vi "TDC_DAQV20_muon.vi"(8 "error in (no error)":errorcluster, 9 "stop":bool=TRUE, 10 "save data":bool=TRUE, 11 "SMA mode":bool=TRUE) -> (3 "rate":dbl)   [LabVIEW 2017]
uses:
  <vilib>/Utility/file.llb/Write Delimited Spreadsheet (DBL).vi
  <vilib>/Utility/file.llb/Write Delimited Spreadsheet (I64).vi
panel:
  out "substring 3":string
  out "hex integer string":string
  out "Year":string
  out "substring 2":string
  out "error out 3":errorcluster
  out "substring":string
  in  "factor":i32=128
  in  "displayCR":bool=TRUE
  in  "Counter Setting":dbl=100000.0 format="%#_13g"
  in  "replace dat":bool
  in  "append csv":bool=TRUE
  out "concatenated string":string
  out "number":u32=23
  out "element":string
  out "fine":u64=375 format="%x"
  in  "UDP Config":bool=TRUE
  in  "data  path":path=path "G:/tdc/2017"
  out "cal 2":u64[](graph)
  in  "Thresholds (mV)":u16[](array[numeric])=[580, 580, 580, 580, 600, 600, 600, 600, 580, 580, 600, 600, 600, 600, 600, 600, 580, 580, 600, 600, 600, 600, 600, 600, 580, 580, 600, 600, 600, 600, 600, 600]
  out "error out 2":errorcluster={"status"=TRUE, "code"=1, "source"="Dequeue Element in TDC_DAQV18_NewStructure.vi"}
  in  "display":bool=TRUE
  in  "Thresholds":u16=580
  in  "one key for threshold":bool=TRUE
  in  "RST":bool
  in  "通道数量":i32=64
  out "Cal Table":u32[](array[numeric])
  in  "channel for cal":i32
  out "channel number":u64
  in  "bytes to read":i32=320
  out "Calibration Counter":i32=100000
  out "Event index":i32=97959
  out "cal":u32[](graph)
  out "error out":errorcluster
  out "appended path":path=path "G:/tdc/2017/test_20240612_084516.dat"
  in  "filename":string="test"
  in  "Events":i32=110000 min=1
  in  "timeout (ms)":i32=10000
  in  "address":string="192.168.10.23"
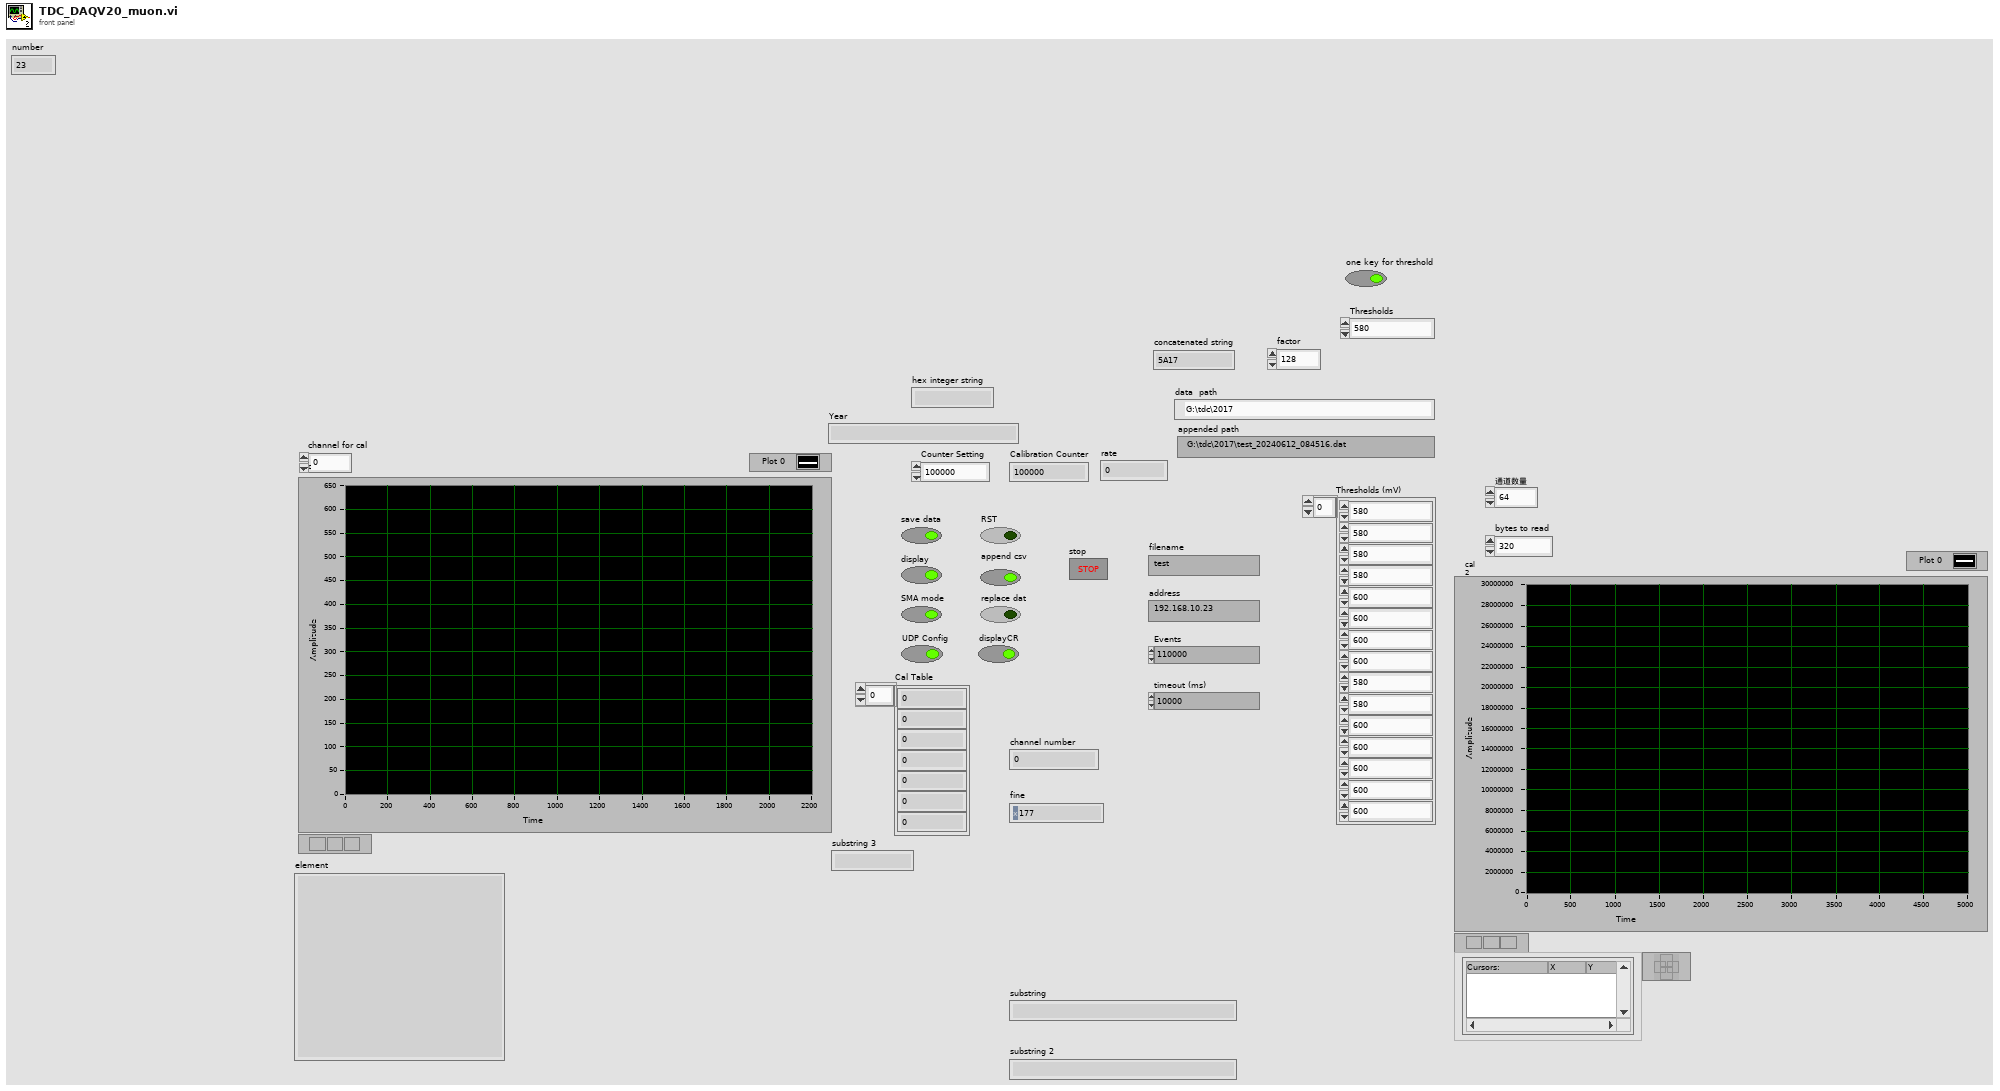
[diagram p1: front panel]
types:
  T1 = enum16{"open", "replace", "create", "open or create", "replace or create", "replace or create with confirmation"}
  T2 = enum16{"Standard", "Buffered", "CRLF", "Immediate"}
  T3 = enum16{"big-endian, network order", "native, host order", "little-endian"}
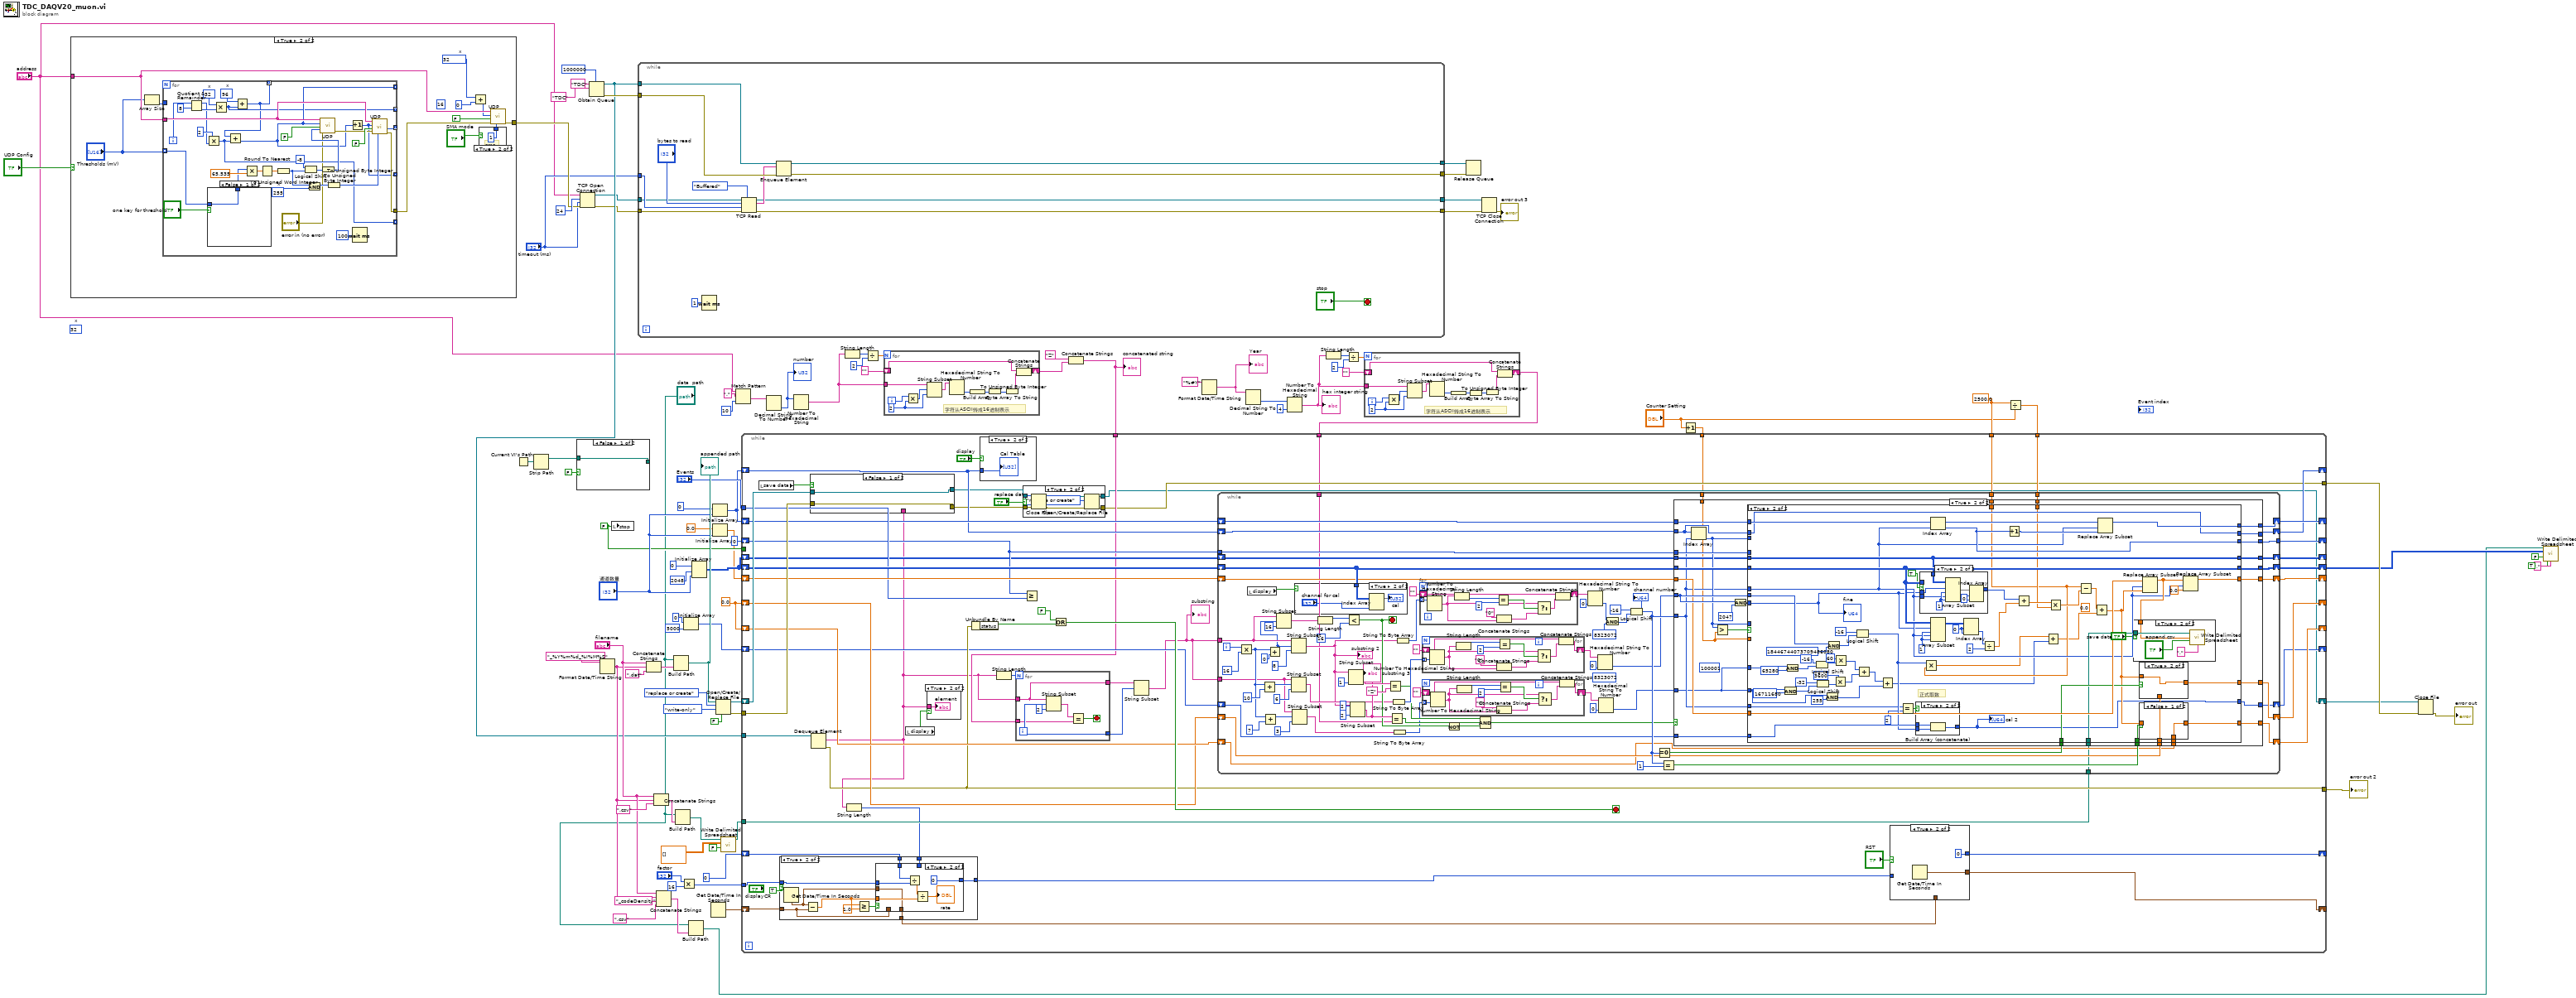
[diagram p0: block diagram]
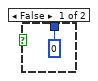
[diagram p3: hidden frame]
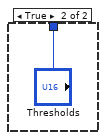
[diagram p4: hidden frame]
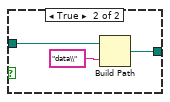
[diagram p5: hidden frame]
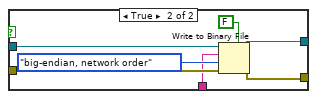
[diagram p7: hidden frame]
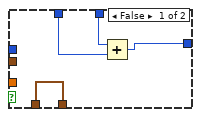
[diagram p10: hidden frame]
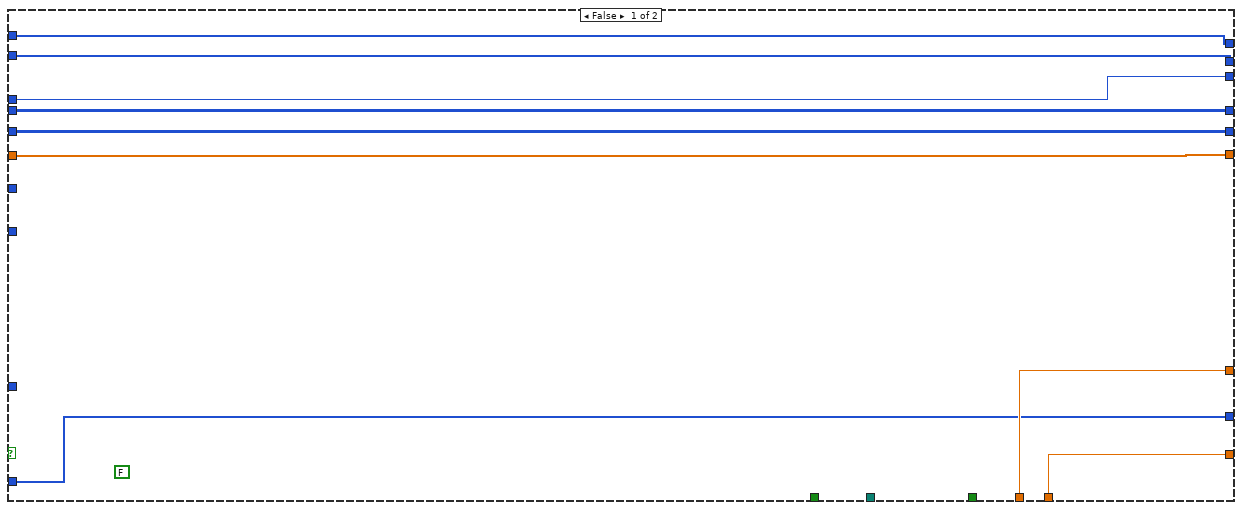
[diagram p14: hidden frame]
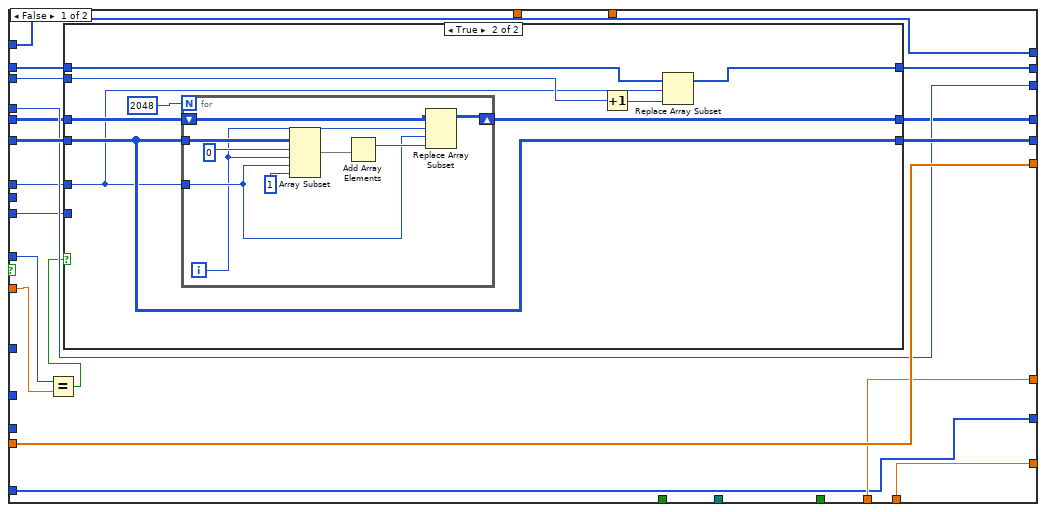
[diagram p15: hidden frame]
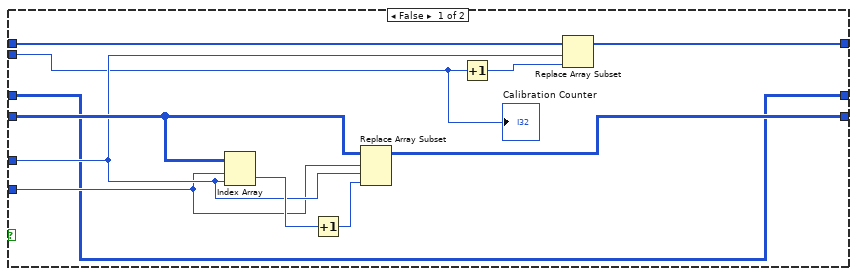
[diagram p16: hidden frame]
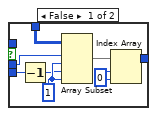
[diagram p19: hidden frame]
diagram:
  w20 = 2500.0 ("x")
  (unwired) u16 32  # x
  w64 = FALSE ("stop")
  w74 = 0.0
  n1 = case shown="True" "UDP Config" {
    tunnel: "address" -> [_ w107]
    tunnel: [_ w104] -> w65
    frame False {
    }
    frame True {
      (unwired) u32 16 ("Address")
      w98 = u16 32  # x
      n2 = Array Size(array="Thresholds (mV)") -> (size(s)=w101:i32)
      n3 = for {
        tunnel: w107 -> [w137]
        tunnel: "Thresholds (mV)" -> [w123] mode=indexing
        tunnel: [w131] -> _ mode=indexing
        tunnel: [w126] -> w105
        tunnel: w101 -> [_]
        tunnel: [w117] -> _ mode=indexing
        tunnel: [w116] -> _ mode=indexing
        tunnel: [w115] -> _ mode=indexing
        tunnel: [w114] -> _ mode=indexing
        tunnel: [w113] -> _ mode=indexing
        i -> [w118]
        w119 = u16 96  # x
        w120 = u16 32  # x
        w133 = u16 255  # x
        n4 = Quotient & Remainder(x=w118, y=8) -> (x-y*floor(x/y)=w112:i32, floor(x/y)=w121:i32)
        n5 = Multiply(x=2, y=w112) -> (x*y=w113:i32)
        n6 = case shown="False" "one key for threshold" {
          tunnel: [w143 "Thresholds"] -> w124
          tunnel: w123 -> [w143 _]
          frame False {
          }
          frame True {
          }
        }
        n7 = Multiply(x=w120, y=w121) -> (x*y=w115:i32)
        n8 = Add(x=w119, y=w115) -> (x+y=w114:i32)
        n9 = Add(x=w114, y=w113) -> (x+y=w117:i32)
        n10 = Multiply(x=w124, y=65.535) -> (x*y=w140:dbl)
        n11 = Round To Nearest(number=w140) -> (nearest integer value=w138:dbl)
        n12 = To Unsigned Word Integer(number=w138) -> (unsigned 16bit integer=w128:u16)
        n13 = Logical Shift(y=i16 -8, x=w128) -> (x << y=w135:u16)
        n14 = And(x=w128, y=w133) -> (x .and. y?=w132:u16)
        n15 = To Unsigned Byte Integer(number=w135) -> (unsigned 8bit integer=w134:u8)
        n16 = call "UDP.vi"("In"=w134, "error in (no error)"="error in (no error)", "Read (TRUE)"=FALSE, "Address"=w117, "IP address"=w137) -> ("error out"=w127:errorcluster)  [unwired: 4 in, 1 out]
        n17 = To Unsigned Byte Integer(number=w132) -> (unsigned 8bit integer=w130:u8)
        n18 = Increment(x=w117) -> (x+1=w116:i32)
        n19 = Wait (ms)(milliseconds to wait=u32 100) -> ()  [unwired: 1 out]
        n20 = call "UDP.vi"("In"=w130, "error in (no error)"=w127, "Read (TRUE)"=FALSE, "Address"=w116, "IP address"=w137) -> ("error out"=w126:errorcluster, "Out"=w131:u8)  [unwired: 4 in]
      }
      n21 = Add(x=w98, y=u32 0 ("Address")) -> (x+y=w97:u32)
      n22 = case shown="True" "SMA mode" {
        tunnel: [u8 0 ("In") u8 1 ("In")] -> w103
        frame False {
        }
        frame True {
          # "sma"
        }
      }
      n23 = call "UDP.vi"("In"=w103, "error in (no error)"=w105, "Read (TRUE)"=FALSE, "Address"=w97, "IP address"=w107) -> ("error out"=w104:errorcluster)  [unwired: 4 in, 1 out]
    }
  }
  n24 = Current VI's Path() -> (path=w90:path)
  n25 = Strip Path(path=w90) -> (stripped path=w89:path)  [unwired: 1 out]
  n26 = case shown="False" FALSE {
    tunnel: w89 -> [w145 w147]
    tunnel: [w145 w146] -> _
    frame False {
    }
    frame True {
      n27 = Build Path(base path=w147, name or relative path="data\\") -> (appended path=w146:path)
    }
  }
  n28 = TCP Open Connection(address="address", remote port or service name=u16 24 ("port"), timeout ms (60000)="timeout (ms)", error in (no error)=w65) -> (connection ID=w48:refnum<k5>, error out=w49:errorcluster)  [unwired: 1 in]
  n29 = Obtain Queue(max queue size (-1, unlimited)=1000000, name (unnamed)="TDC", element data type="TDC" ("name (unnamed)")) -> (queue out=w50:refnum<queue>, error out=w51:errorcluster)  [unwired: 2 in, 1 out]
  n30 = Format Date/Time String(time format string (%c)="_%Y%m%d_%I%M%S") -> (date/time string=w62:string)  [unwired: 2 in]
  n31 = local write "stop"(w64) -> ()
  n32 = while {
    tunnel: w50 -> [w162]
    tunnel: w51 -> [w161]
    tunnel: w49 -> [w159]
    tunnel: "timeout (ms)" -> [w158]
    tunnel: w48 -> [w157]
    tunnel: [w155] -> w47
    tunnel: [w154] -> w46
    tunnel: [w152] -> w45
    tunnel: [w151] -> w44
    stop <- "stop" stop-if-true
    n33 = Wait (ms)(milliseconds to wait=u32 1) -> ()  [unwired: 1 out]
    n34 = TCP Read(connection ID=w157, bytes to read="bytes to read", error in (no error)=w159, 7:T2."Buffered" ("mode (standard)"), 9:w158) -> (connection ID out=w155:refnum<k5>, data out=w156:string, error out=w154:errorcluster)
    n35 = Enqueue Element(queue=w162, element=w156, error in (no error)=w161) -> (queue out=w152:refnum<queue>, error out=w151:errorcluster)  [unwired: 1 in, 1 out]
  }
  n36 = Concatenate Strings("filename", w62, ".dat") -> (w88:string)
  n37 = Concatenate Strings("filename", w62, ".csv") -> (w76:string)
  n38 = Concatenate Strings("filename", w62, "_codeDensity" ("string"), ".csv") -> (w59:string)
  n39 = Build Path(base path="data  path", name or relative path=w88) -> (appended path=w87:path)
  "appended path" <- w87
  n40 = Build Path(base path="data  path", name or relative path=w76) -> (appended path=w71:path)
  n41 = Multiply(x="factor", y=16) -> (x*y=w13:i32)
  n42 = Initialize Array(u32 0 ("element"), 5000 ("dimension size")) -> (w38:u32[])
  n43 = Build Path(base path="data  path", name or relative path=w59) -> (appended path=w56:path)
  n44 = Initialize Array(u32 0 ("element"), 2048 ("dimension size"), "通道数量") -> (w73:u32[][])
  n45 = Get Date/Time In Seconds() -> (seconds since 1Jan1904=w66:timestamp)
  n46 = Initialize Array(u32 0 ("element"), "通道数量") -> (w75:u32[])
  n47 = Initialize Array(0.0, "通道数量") -> (w40:dbl[])
  n48 = Open/Create/Replace File(file path (use dialog)=w87, operation (0:open)=T1."replace or create", access (0:read/write)=enum16{"read/write", "read-only", "write-only"}."write-only", disable buffering (F)=FALSE) -> (refnum out=w92:refnum<file>, error out=w91:errorcluster)  [unwired: 2 in, 1 out]
  n49 = call-poly <vilib>:"Write Delimited Spreadsheet.vi"("file path (dialog if empty)"=w71, "2D data"=dbl[][] [], "append to file? (new file:F)"=FALSE) -> ("new file path (Not A Path if cancelled)"=w70:path)  [unwired: 11 in, 1 out]
  n50 = Match Pattern(string="address", regular expression="." ("search string"), offset (0)=10) -> (after substring=w27:string)  [unwired: 3 out]
  n51 = Decimal String To Number(string=w27) -> (number=w26:i32)  [unwired: 2 in, 1 out]
  "number" <- w26
  n52 = Number To Hexadecimal String(2:w26) -> (0:w24:string)  [unwired: 1 in]
  n53 = String Length(string=w24) -> (length=w32:i32)
  n54 = Divide(x=w32, y=2) -> (x/y=w33:dbl)
  n55 = for {
    N: w33 -> [_]
    shift-right: [w173] -> w23
    shift-left: "" ("format string") -> [w172]
    tunnel: w24 -> [w163]
    i -> [w171]
    w165 = 2 ("y")
    # "字符从ASCII转成16进制表示"
    n56 = Multiply(x=w171, y=w165) -> (x*y=w164:i32)
    n57 = String Subset(string=w163, offset (0)=w164, length (rest)=w165) -> (substring=w166:string)
    n58 = Hexadecimal String To Number(string=w166) -> (number=w170:u32)  [unwired: 2 in, 1 out]
    n59 = Build Array(w170) -> (w169:u32[])
    n60 = To Unsigned Byte Integer(number=w169) -> (unsigned 8bit integer=w168:u8[])
    n61 = Byte Array To String(unsigned byte array=w168) -> (string=w167:string)
    n62 = Concatenate Strings(w172, w167) -> (w173:string)
  }
  n63 = Concatenate Strings("Z", w23) -> (w22:string)
  "concatenated string" <- w22
  n64 = Format Date/Time String(time format string (%c)="%#Y") -> (date/time string=w9:string)  [unwired: 2 in]
  "Year" <- w9
  n65 = Decimal String To Number(string=w9) -> (number=w8:i32)  [unwired: 2 in, 1 out]
  n66 = Number To Hexadecimal String(1:i16 4 ("width (-)"), 2:w8) -> (0:w2:string)
  "hex integer string" <- w2
  n67 = String Length(string=w2) -> (length=w4:i32)
  n68 = Divide(x=w4, y=2) -> (x/y=w5:dbl)
  n69 = for {
    N: w5 -> [_]
    shift-right: [w184] -> w1
    shift-left: "" ("format string") -> [w183]
    tunnel: w2 -> [w174]
    i -> [w182]
    w176 = 2 ("y")
    # "字符从ASCII转成16进制表示"
    n70 = Multiply(x=w182, y=w176) -> (x*y=w175:i32)
    n71 = String Subset(string=w174, offset (0)=w175, length (rest)=w176) -> (substring=w177:string)
    n72 = Hexadecimal String To Number(string=w177) -> (number=w181:u32)  [unwired: 2 in, 1 out]
    n73 = Build Array(w181) -> (w180:u32[])
    n74 = To Unsigned Byte Integer(number=w180) -> (unsigned 8bit integer=w179:u8[])
    n75 = Byte Array To String(unsigned byte array=w179) -> (string=w178:string)
    n76 = Concatenate Strings(w183, w178) -> (w184:string)
  }
  n77 = Release Queue(queue=w45, error in (no error)=w44) -> ()  [unwired: 1 in, 3 out]
  n78 = TCP Close Connection(connection ID=w47, error in (no error)=w46) -> (error out=→"error out 3":errorcluster)  [unwired: 1 in, 1 out]
  n79 = Increment(x="Counter Setting") -> (x+1=w16:dbl)
  n80 = Divide(x=w20, y="Counter Setting") -> (x/y=w19:dbl)
  n81 = while {
    tunnel: w91 -> [w239]
    tunnel: [w213] -> w43
    tunnel: [w197] -> w84
    shift-right: [w236] -> w57
    shift-left: w73 -> [w237]
    shift-right: [w222] -> _
    shift-left: w40 -> [w235]
    tunnel: "Events" -> [w233]
    shift-right: [w232] -> _
    shift-left: w75 -> [w231]
    shift-right: [w230] -> _
    shift-left: u32 0 ("element") -> [w229]
    shift-right: [w228] -> _
    shift-left: w75 -> [w215]
    shift-right: [w227] -> _
    shift-left: w74 -> [w224]
    shift-right: [w226] -> _
    shift-left: w74 -> [w225]
    shift-right: [w217] -> _
    shift-left: w73 -> [w223]
    tunnel: w70 -> [w209]
    shift-right: [w221] -> _
    shift-left: 0 -> [w191]
    shift-right: [w219] -> _
    shift-left: w66 -> [w218]
    tunnel: w64 -> [_]
    tunnel: w50 -> [w214]
    shift-right: [w210] -> _
    shift-left: w38 -> [w211]
    tunnel: w22 -> [w205]
    tunnel: w20 -> [w203]
    tunnel: w19 -> [w202]
    shift-right: [w196] -> w18
    shift-left: w92 -> [w238]
    tunnel: w16 -> [w195]
    tunnel: w13 -> [w188]
    tunnel: w1 -> [w185]
    stop <- w234 stop-if-true
    n82 = local read "save data"() -> (w190:bool)
    n83 = Dequeue Element(queue=w214) -> (element=w201:string, error out=w213:errorcluster)  [unwired: 2 in, 2 out]
    n84 = case shown="False" w190 {
      tunnel: w239 -> [w241 w249]
      tunnel: w238 -> [w242 w248]
      tunnel: w201 -> [_ w245]
      tunnel: [w242 w244] -> w200
      tunnel: [w241 w243] -> w198
      frame False {
      }
      frame True {
        n85 = Write to Binary File(file (use dialog)=w248, data=w245, error in=w249, 5:FALSE ("prepend array or string size? (T)"), 9:T3."big-endian, network order" ("byte order (0:big-endian, network order)")) -> (refnum out=w244:refnum<file>, error out=w243:errorcluster)  [unwired: 1 in, 1 out]
      }
    }
    n86 = String Length(string=w201) -> (length=w192:i32)
    n87 = case shown="True" TRUE {
      tunnel: w218 -> [w266 w271]
      tunnel: [w266 w272] -> w194
      tunnel: w191 -> [w265 w270]
      tunnel: w192 -> [_ w269]
      tunnel: [w265 w268] -> w193
      tunnel: w188 -> [_ w267]
      frame False {
      }
      frame True {
        n88 = Get Date/Time In Seconds() -> (seconds since 1Jan1904=w273:timestamp)
        n89 = Subtract(x=w273, y=w271) -> (x-y=w275:dbl)
        n90 = Greater Or Equal?(x=w275, y=1.0) -> (x >= y?=w276:bool)
        n91 = case shown="True" w276 {
          tunnel: w275 -> [_ w287]
          tunnel: w273 -> [_ w285]
          tunnel: [w280 w285] -> w272
          tunnel: w271 -> [w280 _]
          tunnel: w270 -> [w279 w282]
          tunnel: w269 -> [w278 _]
          tunnel: [w277 0] -> w268
          tunnel: w267 -> [_ w281]
          frame False {
            n92 = Add(x=w278, y=w279) -> (x+y=w277:i32)
          }
          frame True {
            n93 = Divide(x=w282, y=w281) -> (x/y=w284:dbl)
            n94 = Divide(x=w284, y=w287) -> (x/y=→"rate":dbl)
          }
        }
      }
    }
    n95 = local read "display"() -> (w189:bool)
    n96 = case shown="True" w189 {
      tunnel: w201 -> [_ w240]
      frame False {
      }
      frame True {
        "element" <- w240
      }
    }
    n97 = Unbundle By Name(w213) -> ("status"=w212:bool)
    n98 = case shown="True" "display" {
      tunnel: w215 -> [_ w288]
      frame False {
      }
      frame True {
        "Cal Table" <- w288
      }
    }
    n99 = String Length(string=w201) -> (length=w208:i32)
    n100 = for {
      N: w208 -> [_]
      tunnel: w201 -> [w261]
      tunnel: [w261] -> w207
      tunnel: [w260] -> w206
      tunnel: w205 -> [w259]
      i -> [w260]
      stop <- w262 stop-if-true
      n101 = String Subset(string=w261, offset (0)=w260, length (rest)=2 ("length (rest)")) -> (substring=w263:string)
      n102 = Equal?(x=w263, y=w259) -> (x = y?=w262:bool)
    }
    n103 = case shown="True" "replace dat" {
      tunnel: w200 -> [w251 w257]
      tunnel: [w251 w256] -> w196
      tunnel: w198 -> [w250 w253]
      tunnel: [w250 w252] -> w197
      frame False {
      }
      frame True {
        n104 = Close File(refnum=w257, error in=w253) -> (path=w258:path, error out=w254:errorcluster)
        n105 = Open/Create/Replace File(file path (use dialog)=w258, error in=w254, operation (0:open)=T1."replace or create") -> (refnum out=w256:refnum<file>, error out=w252:errorcluster)  [unwired: 3 in, 1 out]
      }
    }
    n106 = Greater Or Equal?(x=w229, y=w233) -> ()  [unwired: 1 out]
    n107 = Or(x=FALSE, y=w212) -> (x .or. y?=w234:bool)
    n108 = String Subset(string=w207, offset (0)=w206) -> (substring=w186:string)  [unwired: 1 in]
    "substring" <- w186
    n109 = while {
      tunnel: w186 -> [w315]
      shift-right: [w366] -> w236
      shift-left: w237 -> [w364]
      shift-right: [w362] -> w222
      shift-left: w235 -> [w363]
      shift-right: [w357] -> w232
      shift-left: w231 -> [w356]
      tunnel: [w355] -> w230
      tunnel: w229 -> [w354]
      shift-right: [w352] -> w228
      shift-left: w215 -> [w353]
      shift-right: [w347] -> w227
      shift-left: w224 -> [w345]
      shift-right: [w343] -> w226
      shift-left: w225 -> [w344]
      tunnel: w209 -> [w342]
      shift-right: [w341] -> w217
      shift-left: w223 -> [w309]
      shift-right: [w338] -> w210
      shift-left: w211 -> [w339]
      tunnel: w186 -> [w301]
      tunnel: w203 -> [w317]
      tunnel: w202 -> [w316]
      tunnel: w195 -> [w308]
      tunnel: w185 -> [w293]
      i -> [w367]
      stop <- w311 stop-if-true
      (unwired) u64 8323072 ("port")
      n110 = Multiply(x=w367, y=16 ("length (rest)")) -> (x*y=w302:i32)
      n111 = local read "display"() -> (w340:bool)
      n112 = Add(x=w302, y=10 ("length (rest)")) -> (x+y=w330:i32)
      n113 = Add(x=w302, y=7 ("length (rest)")) -> (x+y=w304:i32)
      n114 = Add(x=w302, y=0 ("length (rest)")) -> (x+y=w314:i32)
      n115 = String Subset(string=w315, offset (0)=w314, length (rest)=16 ("y")) -> (substring=w312:string)
      n116 = String Subset(string=w315, offset (0)=w314, length (rest)=8 ("length (rest)")) -> (substring=w294:string)
      "substring 2" <- w294
      n117 = String Subset(string=w301, offset (0)=w330, length (rest)=6 ("length (rest)")) -> (substring=w307:string)
      n118 = String Subset(string=w301, offset (0)=w304, length (rest)=3 ("length (rest)")) -> (substring=w297:string)
      n119 = case shown="True" w340 {
        tunnel: w364 -> [_ w393]
        frame False {
        }
        frame True {
          n120 = Index Array(array=w393, index (col)="channel for cal") -> (element=→"cal":u32[])  [unwired: 1 in]
        }
      }
      n121 = String Length(string=w312) -> (length=w361:i32)
      n122 = Less?(x=w361, y=16) -> (x < y?=w311:bool)
      n123 = String Subset(string=w294, length (rest)=1 ("length (rest)")) -> (substring=w335:string)  [unwired: 1 in]
      n124 = String Subset(string=w294, offset (0)=2, length (rest)=2 ("length (rest)")) -> (substring=w318:string)
      "substring 3" <- w318
      n125 = Equal?(x=w335, y="Z" ("format string")) -> (x = y?=w320:bool)
      n126 = Equal?(x=w318, y=w293) -> (x = y?=w319:bool)
      n127 = String To Byte Array(string=w307) -> (unsigned byte array=w327:u8[])
      n128 = String To Byte Array(string=w297) -> (unsigned byte array=w296:u8[])
      n129 = String To Byte Array(string=w294) -> (unsigned byte array=w369:u8[])
      n130 = for {
        shift-right: [w581] -> w324
        shift-left: "" ("format string") -> [w578]
        tunnel: w369 -> [w582] mode=indexing
        n131 = Number To Hexadecimal String(2:w582) -> (0:w574:string)  [unwired: 1 in]
        n132 = String Length(string=w574) -> (length=w580:i32)
        n133 = Equal?(x=w580, y=2) -> (x = y?=w577:bool)
        n134 = Concatenate Strings("0" ("format string"), w574) -> (w576:string)
        n135 = Select(t=w574, s=w577, f=w576) -> (s? t:f=w573:string)
        n136 = Concatenate Strings(w578, w573) -> (w581:string)
      }
      n137 = for {
        shift-right: [w389] -> w325
        shift-left: "" ("format string") -> [w381]
        tunnel: w327 -> [w390] mode=indexing
        n138 = Number To Hexadecimal String(2:w390) -> (0:w383:string)  [unwired: 1 in]
        n139 = String Length(string=w383) -> (length=w388:i32)
        n140 = Concatenate Strings("0" ("format string"), w383) -> (w385:string)
        n141 = Equal?(x=w388, y=2) -> (x = y?=w386:bool)
        n142 = Select(t=w383, s=w386, f=w385) -> (s? t:f=w382:string)
        n143 = Concatenate Strings(w381, w382) -> (w389:string)
      }
      n144 = for {
        shift-right: [w379] -> w300
        shift-left: "" ("format string") -> [w371]
        tunnel: w296 -> [w380] mode=indexing
        n145 = Number To Hexadecimal String(2:w380) -> (0:w373:string)  [unwired: 1 in]
        n146 = String Length(string=w373) -> (length=w378:i32)
        n147 = Concatenate Strings("0" ("format string"), w373) -> (w375:string)
        n148 = Equal?(x=w378, y=2) -> (x = y?=w376:bool)
        n149 = Select(t=w373, s=w376, f=w375) -> (s? t:f=w372:string)
        n150 = Concatenate Strings(w371, w372) -> (w379:string)
      }
      n151 = Not(x=w311) -> (.not. x?=w310:bool)
      n152 = Compound Arithmetic op=AND(w320, w319, w310) -> (w333:bool)
      n153 = Hexadecimal String To Number(string=w324, default (0uL)=u64 0 ("default (0 U32)")) -> (number=w365:u64)  [unwired: 1 in, 1 out]
      n154 = Hexadecimal String To Number(string=w325, default (0uL)=u64 0 ("default (0 U32)")) -> (number=w323:u64)  [unwired: 1 in, 1 out]
      n155 = Hexadecimal String To Number(string=w300, default (0uL)=u64 0 ("default (0 U32)")) -> (number=w295:u64)  [unwired: 1 in, 1 out]
      n156 = And(x=w365, y=u64 8323072 ("port")) -> (x .and. y?=w358:u64)
      n157 = Logical Shift(y=i16 -16, x=w358) -> (x << y=w350:u64)
      "channel number" <- w350
      n158 = Equal To 0?(x=w350) -> (x = 0?=w348:bool)
      n159 = Equal?(x=w350, y=u64 1) -> (x = y?=w346:bool)
      n160 = case shown="True" w333 {
        tunnel: w323 -> [_ w433]
        tunnel: w354 -> [w399 w423]
        tunnel: w364 -> [w402 w432]
        tunnel: [w402 w431] -> w366
        tunnel: [w401 w428] -> w362
        tunnel: w363 -> [w401 w427]
        tunnel: w350 -> [_ w407]
        tunnel: w356 -> [w400 w426]
        tunnel: [w400 w425] -> w357
        tunnel: [w399 w424] -> w355
        tunnel: w353 -> [w398 w422]
        tunnel: [w398 w421] -> w352
        tunnel: w348 -> [_ w420]
        tunnel: w345 -> [w397 w419]
        tunnel: [w397 w418] -> w347
        tunnel: w346 -> [_ w417]
        tunnel: w344 -> [w396 w416]
        tunnel: [w396 w415] -> w343
        tunnel: w309 -> [w395 w413]
        tunnel: [w395 w412] -> w341
        tunnel: w342 -> [_ w411]
        tunnel: w339 -> [w394 w409]
        tunnel: [w394 w408] -> w338
        tunnel: w317 -> [_ w406]
        tunnel: w316 -> [_ w405]
        tunnel: w308 -> [_ w404]
        tunnel: w295 -> [_ w403]
        frame False {
          (unwired) FALSE
        }
        frame True {
          (unwired) 100001 ("y")
          n161 = Index Array(array=w422, index=w407) -> (element=w414:u32)
          n162 = Greater?(x=w414, y=w404) -> (0:w410:bool)
          n163 = And(x=w433, y=u64 2047 ("port")) -> (x .and. y?=w429:u64)
          n164 = case shown="True" w410 {
            tunnel: w433 -> [_ w545]
            tunnel: w432 -> [w451 w531]
            tunnel: [w450 w531] -> w431
            tunnel: w429 -> [w442 w504]
            tunnel: [w449 w515] -> w428
            tunnel: w427 -> [w449 w538]
            tunnel: w423 -> [w447 _]
            tunnel: w407 -> [w445 w513]
            tunnel: w426 -> [w448 w537]
            tunnel: [w448 w536] -> w425
            tunnel: [w447 w534] -> w424
            tunnel: w414 -> [w443 _]
            tunnel: w422 -> [w446 w533]
            tunnel: [w444 w533] -> w421
            tunnel: w420 -> [_ w526]
            tunnel: w419 -> [w441 w525]
            tunnel: [w441 w524] -> w418
            tunnel: w417 -> [_ w523]
            tunnel: w416 -> [w440 w522]
            tunnel: [w440 w521] -> w415
            tunnel: w414 -> [w438 _]
            tunnel: w404 -> [w435 _]
            tunnel: w413 -> [w437 w517]
            tunnel: [w436 w517] -> w412
            tunnel: w411 -> [_ w516]
            tunnel: w409 -> [w434 w510]
            tunnel: [w434 w508] -> w408
            tunnel: w407 -> [_ w505]
            tunnel: w406 -> [_ w502]
            tunnel: w405 -> [_ w503]
            tunnel: w403 -> [_ w497]
            tunnel: w403 -> [_ w485]
            frame False {
              n165 = Equal?(x=w438, y=w435) -> (x = y?=w439:bool)
              n166 = case shown="True" w439 {
                tunnel: w451 -> [w462 w468]
                tunnel: [w460 w468] -> w450
                tunnel: w446 -> [w458 w466]
                tunnel: w445 -> [w457 w463]
                tunnel: [w455 w465] -> w444
                tunnel: w443 -> [w454 w464]
                tunnel: w442 -> [w453 _]
                tunnel: w437 -> [w452 w470]
                tunnel: [w452 w469] -> w436
                frame False {
                  n167 = Index Array(array=w462, index (row)=w453, index (col)=w457) -> (element=w461:u32)
                  n168 = Increment(x=w461) -> (x+1=w459:u32)
                  n169 = Replace Array Subset(array=w462, new element=w459, index (row)=w453, index (col)=w457) -> (w460:u32[][])
                  n170 = Increment(x=w454) -> (x+1=w456:u32)
                  n171 = Replace Array Subset(array=w458, new element=w456, index=w457) -> (w455:u32[])
                  "Calibration Counter" <- w454
                }
                frame True {
                  n172 = for {
                    N: 2048 -> [_]
                    tunnel: w468 -> [w480]
                    tunnel: w463 -> [w473]
                    shift-right: [w475] -> w469
                    shift-left: w470 -> [w476]
                    i -> [w472]
                    n173 = Array Subset(array=w480, index (row)=0 ("索引"), length (row)=w472, index (col)=w473, length (col)=1 ("长度")) -> (w477:u32[][])
                    n174 = Add Array Elements(numeric array=w477) -> (sum=w474:u32)
                    n175 = Replace Array Subset(array=w476, new element=w474, index (row)=w472, index (col)=w473) -> (w475:u32[][])
                  }
                  n176 = Increment(x=w464) -> (x+1=w467:u32)
                  n177 = Replace Array Subset(array=w466, new element=w467, index=w463) -> (w465:u32[])
                }
              }
            }
            frame True {
              (unwired) 0.0 ("x")
              w528 = 0 ("索引 (行)")
              w530 = 1 ("长度")
              # "正式取数"
              n178 = And(x=w485, y=u64 16711680 ("port")) -> (x .and. y?=w494:u64)
              n179 = And(x=w497, y=u64 65280 ("port")) -> (x .and. y?=w500:u64)
              n180 = Logical Shift(y=i16 -16, x=w500) -> (x << y=w491:u64)
              n181 = Logical Shift(y=i16 -32, x=w494) -> (x << y=w493:u64)
              n182 = And(x=w485, y=u64 255 ("port")) -> (x .and. y?=w484:u64)
              n183 = And(x=w545, y=u64 18446744073709486080 ("port")) -> (x .and. y?=w542:u64)
              n184 = Multiply(x=u64 3600, y=w493) -> (x*y=w488:u64)
              n185 = Multiply(x=u64 60, y=w491) -> (x*y=w489:u64)
              n186 = Logical Shift(y=i16 -16, x=w542) -> (x << y=w509:u64)
              n187 = Add(x=w489, y=w488) -> (x+y=w487:u64)
              n188 = Add(x=w487, y=w484) -> (x+y=w481:u64)
              n189 = Equal?(x=w505, y=u32 2) -> (x = y?=w507:bool)
              n190 = case shown="True" w507 {
                tunnel: w510 -> [w546 w549]
                tunnel: w509 -> [_ w548]
                tunnel: [w546 w547] -> w508
                frame False {
                }
                frame True {
                  n191 = Build Array (concatenate)(w549, w548) -> (w547:u64[])
                }
              }
              "cal 2" <- w508
              n192 = case shown="True" TRUE {
                tunnel: [w556 w564] -> w540
                tunnel: w531 -> [_ _]
                tunnel: w513 -> [w561 w562]
                tunnel: w504 -> [w559 w567]
                tunnel: w517 -> [w560 w568]
                frame False {
                  w555 = 0 ("index (row)")
                  w558 = 1 ("长度")
                  n193 = Decrement(x=w561) -> (x-1=w554:u64)
                  n194 = Array Subset(array=w560, index (row)=w559, length (row)=w558, index (col)=w554, length (col)=w558) -> (w557:u32[][])
                  n195 = Index Array(array=w557, index (row)=w555, index (col)=w555) -> (element=w556:u32)
                }
                frame True {
                  w563 = 0 ("index (row)")
                  w566 = 1 ("长度")
                  n196 = Array Subset(array=w568, index (row)=w567, length (row)=w566, index (col)=w562, length (col)=w566) -> (w565:u32[][])
                  n197 = Index Array(array=w565, index (row)=w563, index (col)=w563) -> (element=w564:u32)
                }
              }
              n198 = Multiply(x=w509, y=w502) -> (x*y=w483:dbl)
              n199 = Index Array(array=w537, index=w513) -> (element=w534:u32)
              n200 = Array Subset(array=w531, index (row)=w504, length (row)=w530, index (col)=w513, length (col)=w530) -> (w529:u32[][])
              n201 = Index Array(array=w529, index (row)=w528, index (col)=w528) -> (element=w527:u32)
              n202 = Divide(x=w527, y=u32 2) -> (x/y=w532:dbl)
              n203 = Increment(x=w534) -> (x+1=w535:u32)
              n204 = Add(x=w540, y=w532) -> (x+y=w539:dbl)
              n205 = Add(x=w483, y=w481) -> (x+y=w482:dbl)
              n206 = Multiply(x=w539, y=w503) -> (x*y=w519:dbl)
              n207 = Subtract(x=w502, y=w519) -> (x-y=w501:dbl)
              n208 = Add(x=w501, y=w482) -> (x+y=w520:dbl)
              n209 = Replace Array Subset(array=w537, new element=w535, index=w513) -> (w536:u32[])
              n210 = case shown="True" w526 {
                tunnel: w520 -> [_ w572]
                tunnel: [w571 w572] -> w524
                tunnel: w525 -> [w571 _]
                frame False {
                }
                frame True {
                }
              }
              n211 = case shown="False" w523 {
                tunnel: [w569 w570] -> w521
                tunnel: w522 -> [w569 _]
                tunnel: w520 -> [_ w570]
                frame False {
                }
                frame True {
                }
              }
              n212 = Replace Array Subset(array=w538, new element=w520, index=w513) -> (w514:dbl[])
              n213 = case shown="True" "save data" {
                tunnel: w516 -> [_ w553]
                tunnel: w514 -> [_ w551]
                frame False {
                }
                frame True {
                  n214 = call-poly <vilib>:"Write Delimited Spreadsheet.vi"("file path (dialog if empty)"=w553, "1D data"=w551, "append to file? (new file:F)"="append csv", "delimiter (\\t)"="," ("delimiter (\\t)")) -> ()  [unwired: 10 in, 2 out]
                }
              }
              n215 = Replace Array Subset(array=w514, new element=0.0 ("new element/subarray"), index=w513) -> (w515:dbl[])
              "fine" <- w504
            }
          }
        }
      }
    }
    n216 = case shown="True" "RST" {
      tunnel: w193 -> [w290 _]
      tunnel: [w290 0] -> w221
      tunnel: [w289 w291] -> w219
      tunnel: w194 -> [w289 _]
      frame False {
      }
      frame True {
        n217 = Get Date/Time In Seconds() -> (seconds since 1Jan1904=w291:timestamp)
      }
    }
  }
  "error out 2" <- w43
  n218 = Close File(refnum=w18, error in=w84) -> (error out=→"error out":errorcluster)  [unwired: 1 out]
  n219 = call-poly <vilib>:"Write Delimited Spreadsheet.vi"("file path (dialog if empty)"=w56, "2D data"=w57, "append to file? (new file:F)"=FALSE, "transpose? (no:F)"=TRUE, "delimiter (\\t)"="," ("delimiter (\\t)")) -> ()  [unwired: 9 in, 2 out]
